vi "LV86_MaskIt.vi"(1 "ROI":cluster{i32, i32, i32, i32}, 2 "Image In":T1 {"Dialogs" format="%.0b"}) -> (0 "Image Out":T1 {"Dialogs" format="%.0b"})   [LabVIEW 2024]
doc: "This VI builds a mask for a Region of Interst on an 8 bit image input."
uses:
  <userlib>/ImageProcessing/QTLIB_2595_LV86/QT_Image.ctl
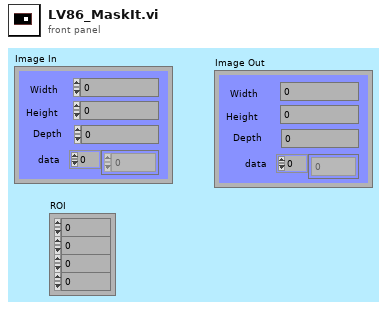
[diagram p1: front panel]
types:
  T1 = typedef "QT_Image.ctl" = cluster{"Width":i32, "Height":i32, "Depth":i32, "data":u8[], "Compressed data":u8[], "Color table":u32[], "Duration":i32, "Options":i32, "Timestamp":i32, "ID":i32, "Reserved":i32, "Dialogs":u32}
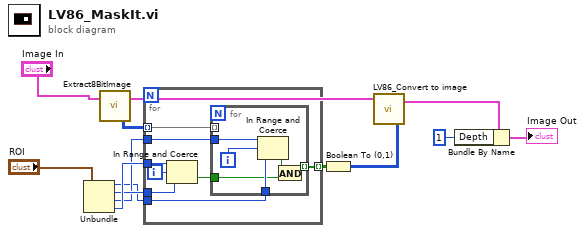
[diagram p0: block diagram]
diagram:
  n1 = Unbundle("ROI") -> (w5:i32, w7:i32, w6:i32, w8:i32)
  n2 = call <userlib>:"Extract8BitImage.vi"("Image in"="Image In") -> ("Intensity Graph"=w11:u8[][], "Image out"=w13:T1)  [unwired: 1 in]
  n3 = for {
    tunnel: w11 -> [w21] mode=indexing
    tunnel: w8 -> [w19]
    tunnel: w7 -> [w18]
    tunnel: w6 -> [w17]
    tunnel: w5 -> [w16]
    tunnel: [w15] -> w9 mode=indexing
    i -> [w20]
    n4 = In Range and Coerce(upper limit=w19, x=w20, lower limit=w18) -> (In Range?=w14:bool)  [unwired: 1 out]
    n5 = for {
      tunnel: w21 -> [_] mode=indexing
      tunnel: w17 -> [w26]
      tunnel: w16 -> [w25]
      tunnel: [w22] -> w15 mode=indexing
      tunnel: w14 -> [w23]
      i -> [w27]
      n6 = In Range and Coerce(upper limit=w26, x=w27, lower limit=w25) -> (In Range?=w24:bool)  [unwired: 1 out]
      n7 = And(x=w24, y=w23) -> (x .and. y?=w22:bool)
    }
  }
  n8 = Boolean To (0,1)(Boolean=w9) -> (0, 1=w4:i16[][])
  n9 = call <userlib>:"LV86_Convert to image.vi"("Intensity Graph"=w4, "Image In"=w13) -> ("Image Out"=w2:T1)  [unwired: 1 in]
  n10 = Bundle By Name(cluster=w2, "Depth"=1) -> (→"Image Out":T1)
